vi "PFI-28000-System_Destroy.vi"(0 "PFI-28000-System in":refnum<class "PFI-28000-System.lvclass">, 11 "error in (no error)":errorcluster) -> (15 "error out":errorcluster)   [LabVIEW 2017, in "PFI-28000-System.lvclass"]
uses:
  PFI-28000-System.lvclass
  C:/wc/07143 Precision Filters 28000 Support/Driver/source/Base/PFI-28000-Base.lvclass
  PFI-28000-System.lvclass/PFI-28000-System.ctl
  Overload/PFI-28000-Overload.lvclass
  Card/PFI-28000-Card.lvclass
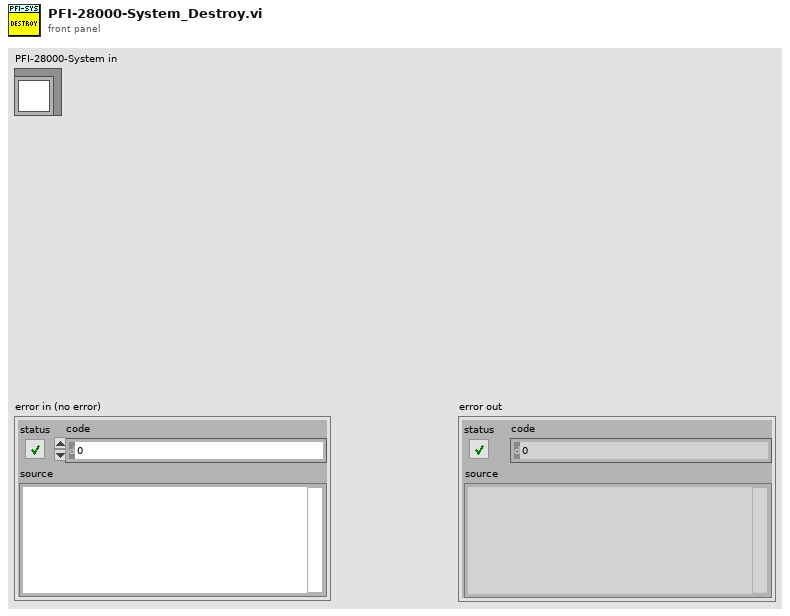
[diagram p1: front panel]
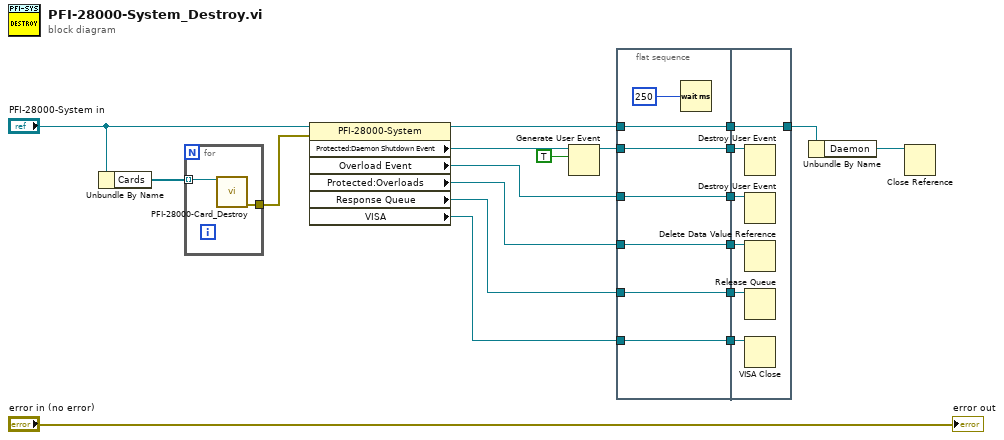
[diagram p0: block diagram]
diagram:
  n1 = Unbundle By Name("PFI-28000-System in") -> ("Cards"=w2:refnum<class "PFI-28000-Card.lvclass">[])
  n2 = for {
    tunnel: w2 -> [w22] mode=indexing
    tunnel: [w21] -> w1
    n3 = call-dynamic "PFI-28000-Card_Destroy.vi"("PFI-28000-Card in"=w22) -> ("error out"=w21:errorcluster)  [unwired: 14 in]
  }
  n4 = property class="PFI-28000-System"(reference="PFI-28000-System in", error in=w1) -> (reference out=w7:refnum<class "PFI-28000-System.lvclass">, "Protected:Daemon Shutdown Event"=w19:refnum<user-event>, "Overload Event"=w15:refnum<user-event>, "Protected:Overloads"=w13:refnum<data-value>, "Response Queue"=w11:refnum<queue>, "VISA"=w9:refnum<visa-resource-name>)  [unwired: 1 out]
  n5 = Generate User Event(user event=w19, event data cluster=TRUE ("event data")) -> (user event out=w16:refnum<user-event>)  [unwired: 2 in, 1 out]
  n6 = flat-sequence {
    tunnel: [w29] -> w17
    tunnel: w16 -> [w29]
    tunnel: w15 -> [w27]
    tunnel: [w27] -> w14
    tunnel: w13 -> [w26]
    tunnel: [w26] -> w12
    tunnel: w11 -> [w25]
    tunnel: [w25] -> w10
    tunnel: w9 -> [w24]
    tunnel: [w24] -> w8
    tunnel: w7 -> [w23]
    tunnel: [w23] -> w6
    tunnel: w17 -> [w35]
    tunnel: w14 -> [w34]
    tunnel: w12 -> [w30]
    tunnel: w10 -> [w33]
    tunnel: w8 -> [w32]
    tunnel: [w31] -> w5
    tunnel: w6 -> [w31]
    frame #0 {
      n7 = Wait (ms)(milliseconds to wait=u32 250) -> ()  [unwired: 1 out]
    }
    frame #1 {
      n8 = Destroy User Event(user event=w35) -> ()  [unwired: 1 in, 1 out]
      n9 = Destroy User Event(user event=w34) -> ()  [unwired: 1 in, 1 out]
      n10 = Delete Data Value Reference(data value reference=w30) -> ()  [unwired: 1 in, 2 out]
      n11 = Release Queue(queue=w33) -> ()  [unwired: 2 in, 3 out]
      n12 = VISA Close(VISA resource name=w32) -> ()  [unwired: 1 in, 1 out]
    }
  }
  n13 = Unbundle By Name(w5) -> ("Daemon"=w4:refnum<vi>)
  n14 = Close Reference(reference=w4) -> ()  [unwired: 1 in, 1 out]
  "error out" <- "error in (no error)"
